vi "Server Panel2.vi"() -> ()   [LabVIEW 2017]
panel:
  out "elapsed ms":u32
  in  "Reader":i32=50000
  in  "Writer":i32=1
  in  "Close":bool
  in  "Writes":bool=TRUE
  in  "String Array 2":string[](array[string])
  in  "Numeric Array 2":dbl[](array[numeric])
  in  "Boolean Array 2":bool[](array[boolean])
  out "String Array":string[](array[string])
  out "Numeric Array":dbl[](array[numeric])
  out "Boolean Array":bool[](array[boolean])
  in  "String 2":string
  in  "Numeric":dbl
  in  "Open":bool
  in  "Reads":bool=TRUE
  in  "ms between":u32
  out "Boolean":bool
  out "String":string
  out "Numeric":dbl
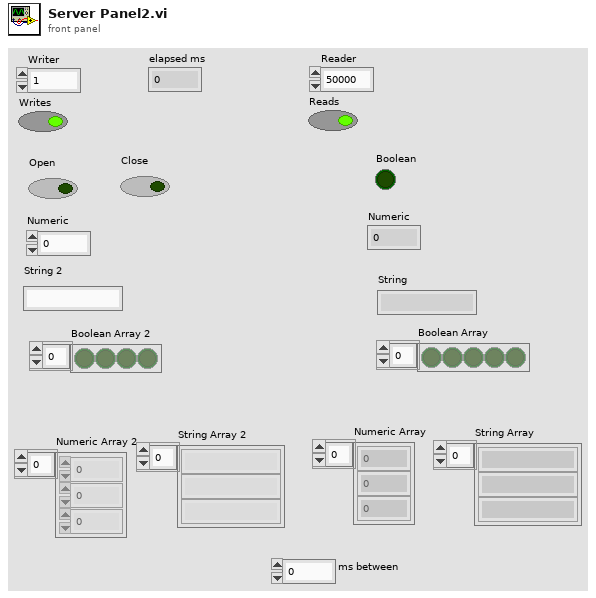
[diagram p1: front panel]
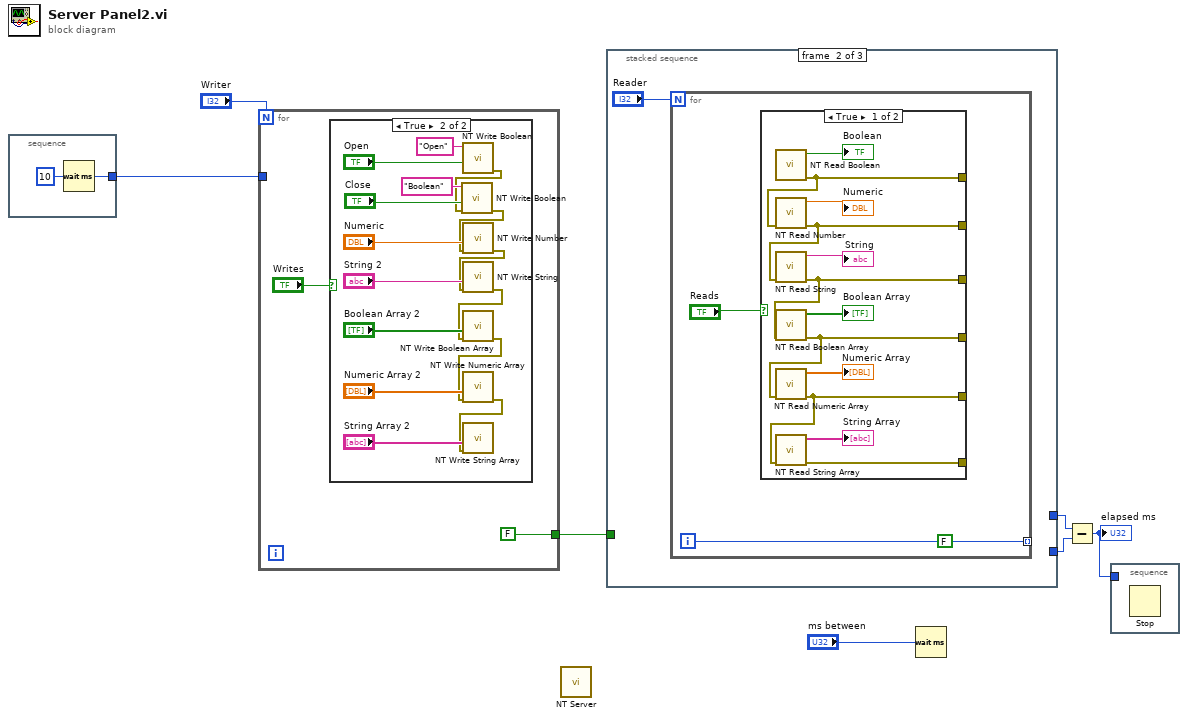
[diagram p0: block diagram]
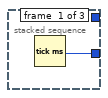
[diagram p3: hidden frame]
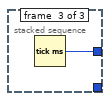
[diagram p5: hidden frame]
diagram:
  n1 = stacked-sequence {
    tunnel: [w8] -> w1
    frame #0 {
      n2 = Wait (ms)(milliseconds to wait=u32 10) -> (millisecond timer value=w8:u32)
    }
  }
  n3 = for {
    N: "Writer" -> [_]
    tunnel: [FALSE] -> w2
    tunnel: w1 -> [_]
    n4 = case shown="True" "Writes" {
      frame False {
      }
      frame True {
        n5 = call <vilib>:"NT Write Boolean.vi"("Boolean"="Open", "Name"="Open") -> ("error out"=w17:errorcluster)  [unwired: 9 in]
        n6 = call <vilib>:"NT Write Boolean.vi"("error in"=w17, "Boolean"="Close", "Name"="Boolean") -> ("error out"=w16:errorcluster)  [unwired: 8 in]
        n7 = call <vilib>:"NT Write Number.vi"("error in"=w16, "Numeric"="Numeric") -> ("error out"=w15:errorcluster)  [unwired: 9 in]
        n8 = call <vilib>:"NT Write String.vi"("error in"=w15, "String"="String 2") -> ("error out"=w14:errorcluster)  [unwired: 9 in]
        n9 = call <vilib>:"NT Write Boolean Array.vi"("error in"=w14, "Boolean Array"="Boolean Array 2") -> ("error out"=w13:errorcluster)  [unwired: 9 in]
        n10 = call <vilib>:"NT Write Numeric Array.vi"("error in"=w13, "Numeric Array"="Numeric Array 2") -> ("error out"=w12:errorcluster)  [unwired: 9 in]
        n11 = call <vilib>:"NT Write String Array.vi"("error in"=w12, "String Array"="String Array 2") -> ()  [unwired: 9 in, 1 out]
      }
    }
  }
  n12 = call <vilib>:"NT Server.vi"() -> ()  [unwired: 12 in]
  n13 = stacked-sequence {
    tunnel: [w27 _ _] -> w7
    tunnel: [_ _ w43] -> w6
    tunnel: w2 -> [_ _ _]
    frame #0 {
      n14 = Tick Count (ms)() -> (millisecond timer value=w27:u32)
    }
    frame #1 {
      n15 = for {
        N: "Reader" -> [_]
        tunnel: [w29] -> _ mode=indexing
        i -> [w29]
        (unwired) FALSE
        n16 = case shown="True" "Reads" {
          tunnel: [w35 _] -> _
          tunnel: [w33 _] -> _
          tunnel: [w34 _] -> _
          tunnel: [w36 _] -> _
          tunnel: [w31 _] -> _
          tunnel: [w32 _] -> _
          frame True {
            n17 = call <vilib>:"NT Read Boolean.vi"() -> ("error out"=w35:errorcluster, "Boolean"=→"Boolean":bool)  [unwired: 10 in]
            n18 = call <vilib>:"NT Read Number.vi"("error in"=w35) -> ("error out"=w34:errorcluster, "Numeric"=→"Numeric":dbl)  [unwired: 9 in]
            n19 = call <vilib>:"NT Read String.vi"("error in"=w34) -> ("error out"=w33:errorcluster, "String"=→"String":string)  [unwired: 9 in]
            n20 = call <vilib>:"NT Read Boolean Array.vi"("error in"=w33) -> ("error out"=w32:errorcluster, "Boolean Array"=→"Boolean Array":bool[])  [unwired: 9 in]
            n21 = call <vilib>:"NT Read Numeric Array.vi"("error in"=w32) -> ("error out"=w31:errorcluster, "Numeric Array"=→"Numeric Array":dbl[])  [unwired: 9 in]
            n22 = call <vilib>:"NT Read String Array.vi"("error in"=w31) -> ("error out"=w36:errorcluster, "String Array"=→"String Array":string[])  [unwired: 9 in]
          }
          frame False {
          }
        }
      }
    }
    frame #2 {
      n23 = Tick Count (ms)() -> (millisecond timer value=w43:u32)
    }
  }
  n24 = Wait (ms)(milliseconds to wait="ms between") -> ()  [unwired: 1 out]
  n25 = Subtract(x=w6, y=w7) -> (x-y=w5:u32)
  "elapsed ms" <- w5
  n26 = stacked-sequence {
    tunnel: w5 -> [_]
    frame #0 {
      n27 = Stop() -> ()  [unwired: 1 in]
    }
  }
